vi "Class to Variant.vi"(8 "error in (no error)":errorcluster, 11 "Run VI in":refnum<class "Run VI.lvclass">) -> (0 "error out":errorcluster, 1 "Display":string, 2 "Data":variant, 3 "Run VI out":refnum<class "Run VI.lvclass">)   [LabVIEW 2014, in "Run VI.lvclass"]
uses:
  Run VI.lvclass
  Run VI.lvclass/Run VI.ctl
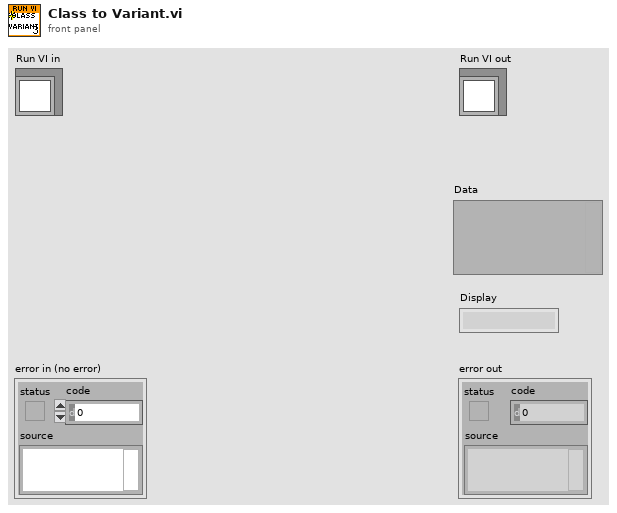
[diagram p1: front panel]
types:
  T1 = typedef "Run VI - STYP.ctl" = cluster{"Executor_Number":string, "VI_Path":string, "Wait_Until_Done":bool}
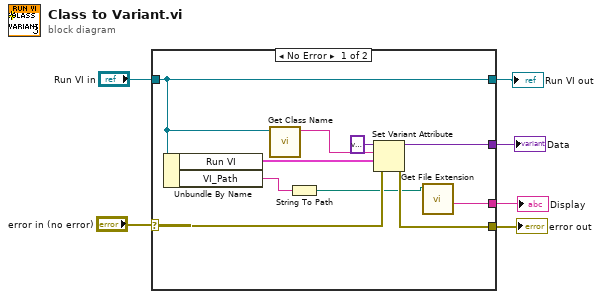
[diagram p0: block diagram]
diagram:
  n1 = case shown="No Error" "error in (no error)" {
    selector: "error in (no error)" -> [w10 w17]
    tunnel: [w13 w18] -> w4
    tunnel: "Run VI in" -> [w13 w18]
    tunnel: [w12 _] -> w3
    tunnel: [w9 w17] -> w2
    tunnel: [w7 _] -> w1
    frame No Error {
      n2 = Unbundle By Name(w13) -> ("Run VI"=w16:T1, "VI_Path"=w11:string)
      n3 = call "Get Class Name.vi"("lvclass"=w13) -> ("Class Name"=w14:string)  [unwired: 10 in]
      n4 = String To Path(string=w11) -> (path=w8:path)
      n5 = Set Variant Attribute(Variant=variant ("variant"), name=w14, value=w16, error in=w10) -> (Variant out=w12:variant, error out=w9:errorcluster)  [unwired: 1 out]
      n6 = call <vilib>:"Get File Extension.vi"("file"=w8) -> ("filename without extension"=w7:string)  [unwired: 7 in, 3 out]
    }
    frame Error {
    }
  }
  "error out" <- w2
  "Run VI out" <- w4
  "Data" <- w3
  "Display" <- w1
